vi "json.pretty_print.vi"(8 "error in":errorcluster, 11 "JSON in":string) -> (0 "error out":errorcluster, 2 "Pretty JSON Out":string)   [LabVIEW 2020, in "Nominal Client.lvclass"]
doc: "Pretty printing JSON formats the data with indentation and line breaks, making it easier to read and debug. While useful for human readability, it increases file size and is not ideal for performance-critical tasks."
uses:
  Nominal Client.lvclass
  <vilib>/JDP Science/JSONtext/JSONtext.lvlib
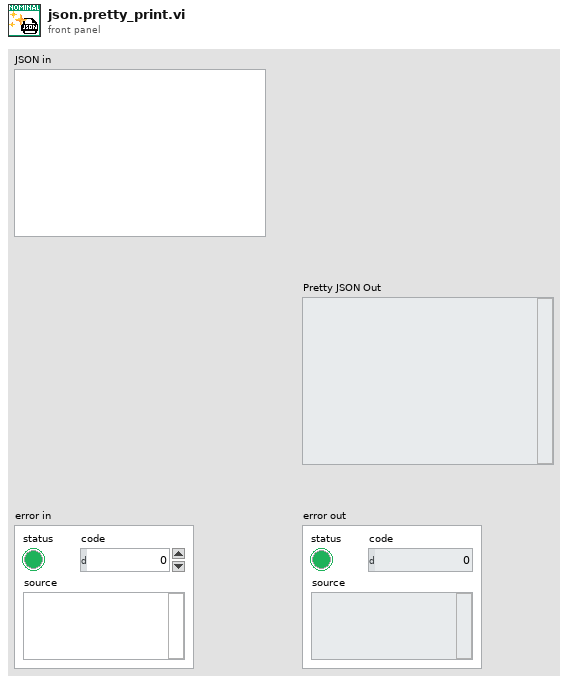
[diagram p1: front panel]
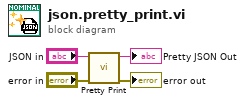
[diagram p0: block diagram]
diagram:
  n1 = call <vilib>:"Pretty Print.vi"("error in (no error)"="error in", "JSON"="JSON in") -> ("error out"=→"error out":errorcluster, "<JSON>"=→"Pretty JSON Out":string)  [unwired: 7 in, 1 out]
